vi "DHE_is_unsc_present.vi"(8 "error in (no error)":errorcluster) -> (0 "error out":errorcluster, 2 "value":bool)   [LabVIEW 2016]
uses:
  DBSHAND/private/vis/DatabaseHand_Element_Get(bool).vi
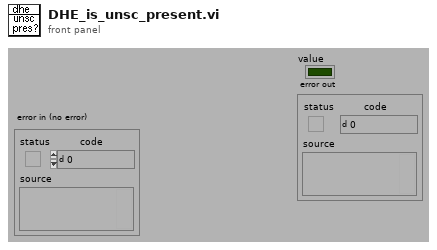
[diagram p1: front panel]
types:
  T1 = typedef "DatabaseHand_RefNum.ctl" = refnum<vi>
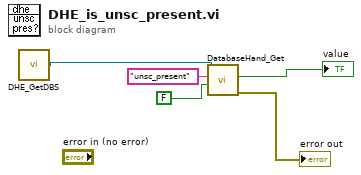
[diagram p0: block diagram]
diagram:
  n1 = call "DHE_GetDBS.vi"() -> ("DHE_DBSRef"=w1:T1)  [unwired: 9 out]
  n2 = call-poly "DatabaseHand_Get.vi"("default value"=FALSE, "name"="unsc_present", "Database RefNum in"=w1) -> ("error out"=→"error out":errorcluster, "value"=→"value":bool)  [unwired: 2 in, 5 out]
